vi "FPGAToHost(Array).vi"(7 "Maximum Pixels per Read":i32=-1, 8 "error in (no error)":errorcluster, 9 "Image in":T1, 10 "Read Timeout (ms)":i32=5000, 11 "Refnum in":refnum<k20>) -> (0 "error out":errorcluster, 2 "Image Out":T1, 3 "Refnum out":refnum<k20>)   [LabVIEW 2016]
uses:
  <vilib>/vision/Image Controls.llb/IMAQ Image.ctl
  <vilib>/vision/EDVR.llb/IMAQ ImageToEDVR 2D U8.vi
  <vilib>/rvi/errors/niLvFpgaAdjustHostInterfaceError.vi
  <vilib>/rvi/interface/nirviMethod/nirviMethod.xnode
  <vilib>/FPGAPlugInAG/Dynamic/niLvFpga_ReadFifo_Dynamic.vi
  <vilib>/rvi/errors/niLvFpgaMergeErrorWithErrorCode.vi
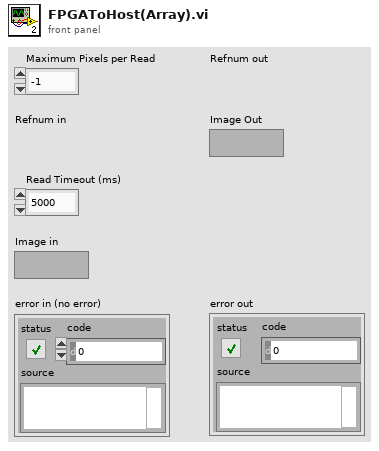
[diagram p1: front panel]
types:
  T1 = typedef "IMAQ Image.ctl" = refnum<image>
  T2 = typedef "Image Type" = u32
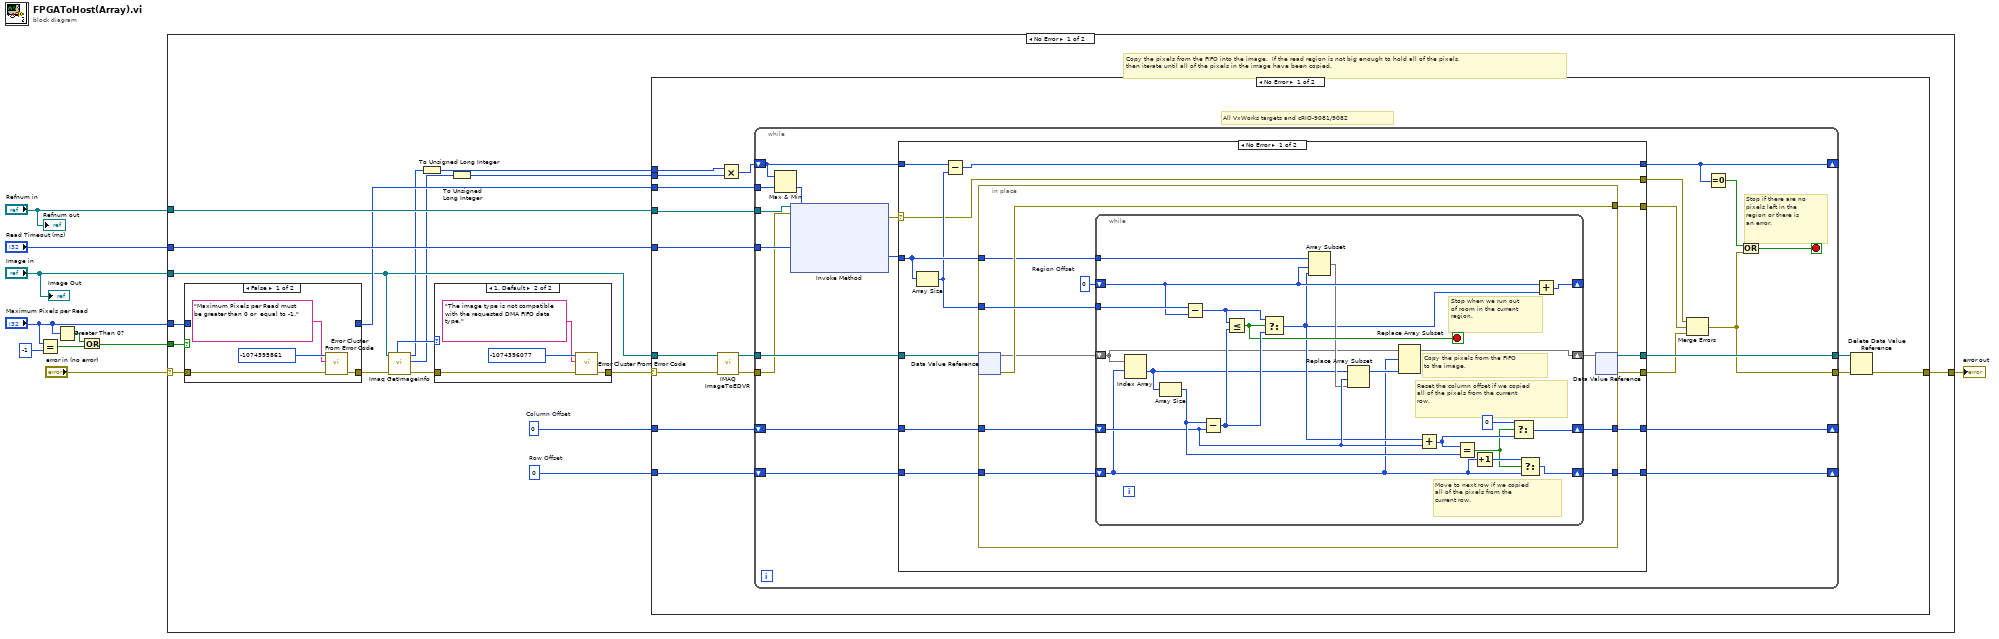
[diagram p0: block diagram]
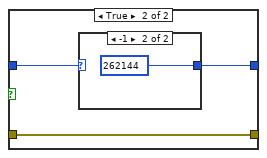
[diagram p2: hidden frame]
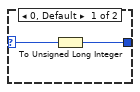
[diagram p3: hidden frame]
diagram:
  n1 = Equal?(x="Maximum Pixels per Read", y=-1) -> (x = y?=w5:bool)
  n2 = Greater Than 0?(x="Maximum Pixels per Read") -> (x > 0?=w4:bool)
  n3 = Or(x=w4, y=w5) -> (x .or. y?=w6:bool)
  n4 = case shown="No Error" "error in (no error)" {
    selector: "error in (no error)" -> [w15 w131]
    tunnel: "Refnum in" -> [w26 _]
    tunnel: "Read Timeout (ms)" -> [w23 _]
    tunnel: w6 -> [w22 _]
    tunnel: "Maximum Pixels per Read" -> [w21 _]
    tunnel: "Image in" -> [w17 _]
    tunnel: [w16 w131] -> w9
    frame No Error {
      w27 = u32 0  # Row Offset
      w28 = u32 0  # Column Offset
      # "Copy the pixels from the FIFO into the image.  If the read region is not big enough to hold all of the pixels,\nthen iterate until all of the pixels in the image have been copied."
      n5 = case shown="False" w22 {
        tunnel: w15 -> [w30 w35]
        tunnel: [w29 w35] -> w20
        tunnel: w21 -> [_ w34]
        tunnel: [_ w33] -> w19
        frame False {
          n6 = call <vilib>:"Error Cluster From Error Code.vi"("error in (no error)"=w30, "error message (\"\")"="Maximum Pixels per Read must be greater than 0 or  equal to -1." ("error message (\"\")"), "error code (0)"=-1074395861) -> ("error out"=w29:errorcluster)  [unwired: 6 in]
        }
        frame True {
          n7 = case shown="-1" w34 {
            selector: w34 -> [w37 _]
            tunnel: [w36 u32 262144 ("Maximum Pixels per Write")] -> w33
            frame 0, Default {
              n8 = To Unsigned Long Integer(number=w37) -> (unsigned 32bit integer=w36:u32)
            }
            frame -1 {
            }
          }
        }
      }
      n9 = call "Imaq GetImageInfo"("error in (no error)"=w20, "Image"=w17) -> ("error out"=w24:errorcluster, "Y Resolution"=w13:i32, "X Resolution"=w14:i32, "Image Type"=w25:T2)  [unwired: 2 in, 4 out]
      n10 = To Unsigned Long Integer(number=w14) -> (unsigned 32bit integer=w12:u32)
      n11 = case shown="1, Default" w25 {
        tunnel: w24 -> [w39 w41]
        tunnel: [w39 w40] -> w18
        frame 0 {
          # "Allowed types are:\nGrayscale (U8)"
        }
        frame 1, Default {
          n12 = call <vilib>:"Error Cluster From Error Code.vi"("error in (no error)"=w41, "error message (\"\")"="The image type is not compatible with the requested DMA FIFO data type." ("error message (\"\")"), "error code (0)"=-1074396077) -> ("error out"=w40:errorcluster)  [unwired: 6 in]
        }
      }
      n13 = To Unsigned Long Integer(number=w13) -> (unsigned 32bit integer=w11:u32)
      n14 = case shown="No Error" w18 {
        selector: w18 -> [w57 w130]
        tunnel: w28 -> [w56 _]
        tunnel: w27 -> [w55 _]
        tunnel: w26 -> [w53 _]
        tunnel: [w51 w130] -> w16
        tunnel: w19 -> [w52 _]
        tunnel: w23 -> [w54 _]
        tunnel: w17 -> [w58 _]
        tunnel: w12 -> [w50 _]
        tunnel: w11 -> [w49 _]
        frame No Error {
          # "All VxWorks targets and cRIO-9081/9082"
          n15 = call-poly <vilib>:"IMAQ ImageToEDVR.vi"("error in (no error)"=w57, "Image"=w58) -> ("error out"=w47:errorcluster, "EDVR 2D U8"=w48:refnum<data-value>)  [unwired: 7 in, 1 out]
          n16 = Multiply(x=w50, y=w49) -> (x*y=w44:u32)
          n17 = while {
            shift-right: [w70] -> _
            shift-left: w44 -> [w66]
            shift-right: [w75] -> _
            shift-left: w56 -> [w77]
            shift-right: [w78] -> _
            shift-left: w55 -> [w76]
            tunnel: w53 -> [w74]
            tunnel: [w72] -> w46
            tunnel: [w68] -> w45
            tunnel: w52 -> [w64]
            tunnel: w54 -> [w63]
            tunnel: w48 -> [w60]
            tunnel: w47 -> [w59]
            stop <- w69 stop-if-true
            # "Stop if there are no\npixels left in the \nregion or there is\nan error."
            n18 = Max & Min(x=w66, y=w64) -> (min(x,y)=w65:u32)  [unwired: 1 out]
            n19 = xnode "Invoke Method"("FPGA VI Reference In"=w74, "error in"=w59, "Number of Elements"=w65, "Timeout (ms)"=w63) -> ("error out"=w73:errorcluster, "Data"=w79:u8[])  [unwired: 2 out]
            n20 = case shown="No Error" w73 {
              selector: w73 -> [w80 w125]
              tunnel: w66 -> [w92 w128]
              tunnel: [w91 w128] -> w70
              tunnel: w60 -> [w90 w129]
              tunnel: w79 -> [w82 _]
              tunnel: [w89 w126] -> w78
              tunnel: w77 -> [w88 w127]
              tunnel: w76 -> [w87 w126]
              tunnel: [w86 w127] -> w75
              tunnel: [w85 w129] -> w72
              tunnel: [w80 w125] -> w62
              tunnel: [w84 _] -> w61
              tunnel: [w83 _] -> w71
              frame No Error {
                n21 = Array Size(array=w82) -> (size(s)=w81:i32)
                n22 = Subtract(x=w92, y=w81) -> (x-y=w91:u32)
                n23 = in-place {
                  in-place-border: w81 -> [w100]
                  in-place-border: [w102] -> w89
                  in-place-border: w88 -> [w99]
                  in-place-border: w87 -> [w95]
                  in-place-border: [w98] -> w86
                  in-place-border: [w97] -> w83
                  in-place-border: w82 -> [w93]
                  w101 = u32 0  # Region Offset
                  n24 = in-place-dvr #1(w90) -> (w96:u8[][], w97:errorcluster)
                  n25 = while {
                    shift-right: [w122] -> _
                    shift-left: w101 -> [w121]
                    tunnel: w93 -> [w111]
                    tunnel: w100 -> [w124]
                    shift-right: [w116] -> w98
                    shift-left: w99 -> [w112]
                    shift-right: [w103] -> w94
                    shift-left: w96 -> [w106]
                    shift-right: [w114] -> w102
                    shift-left: w95 -> [w104]
                    stop <- w113 stop-if-true
                    # "Stop when we run out\nof room in the current\nregion."
                    # "Copy the pixels from the FIFO\nto the image."
                    # "Reset the column offset if we copied\nall of the pixels from the current\nrow."
                    # "Move to next row if we copied\nall of the pixels from the\ncurrent row."
                    n26 = Index Array(array=w106, index (row)=w104) -> (element=w107:u8[])  [unwired: 1 in]
                    n27 = Array Size(array=w107) -> (size(s)=w120:i32)
                    n28 = Subtract(x=w124, y=w121) -> (x-y=w123:u32)
                    n29 = Subtract(x=w120, y=w112) -> (x-y=w119:u32)
                    n30 = Less Or Equal?(x=w123, y=w119) -> (x <= y?=w113:bool)
                    n31 = Select(t=w123, s=w113, f=w119) -> (s? t:f=w109:u32)
                    n32 = Array Subset(array=w111, index=w121, length=w109) -> (w110:u8[])
                    n33 = Replace Array Subset(array=w107, new element=w110, index=w112) -> (w105:u8[])
                    n34 = Replace Array Subset(array=w106, new element=w105, index (row)=w104) -> (w103:u8[][])  [unwired: 1 in]
                    n35 = Add(x=w109, y=w112) -> (x+y=w117:u32)
                    n36 = Equal?(x=w117, y=w120) -> (x = y?=w108:bool)
                    n37 = Increment(x=w104) -> (x+1=w115:u32)
                    n38 = Select(t=u32 0 ("Elements In Region"), s=w108, f=w117) -> (s? t:f=w116:u32)
                    n39 = Select(t=w115, s=w108, f=w104) -> (s? t:f=w114:u32)
                    n40 = Add(x=w121, y=w109) -> (x+y=w122:u32)
                  }
                  n41 = in-place-dvr #1(w94) -> (w85:refnum<data-value>, w84:errorcluster)
                }
              }
              frame Error {
              }
            }
            n42 = Merge Errors(w62, w71, w61) -> (w68:errorcluster)
            n43 = Equal To 0?(x=w70) -> (x = 0?=w67:bool)
            n44 = Or(x=w67, y=w68) -> (x .or. y?=w69:bool)
          }
          n45 = Delete Data Value Reference(data value reference=w46, error in=w45) -> (error out=w51:errorcluster)  [unwired: 1 out]
        }
        frame Error {
        }
      }
    }
    frame Error {
    }
  }
  "error out" <- w9
  "Image Out" <- "Image in"
  "Refnum out" <- "Refnum in"
